vi "Samp.vi"() -> ()   [LabVIEW 2020]
panel:
  out "subarray":dbl[](array[numeric])
  out "Array 2":i32[](array[numeric])
  out "Array":i32[](array[numeric])
  out "x*y":dbl
  out "Waveform Graph":cluster{i32, dbl, i32[]}(graph)
  in  "stop":bool
  out "x":i32
  out "min index(es)":i32
  out "min value":i32
  out "max index(es)":i32
  out "max value":i32
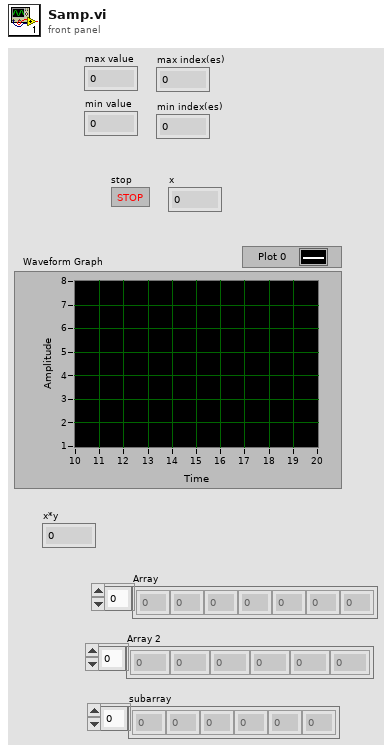
[diagram p1: front panel]
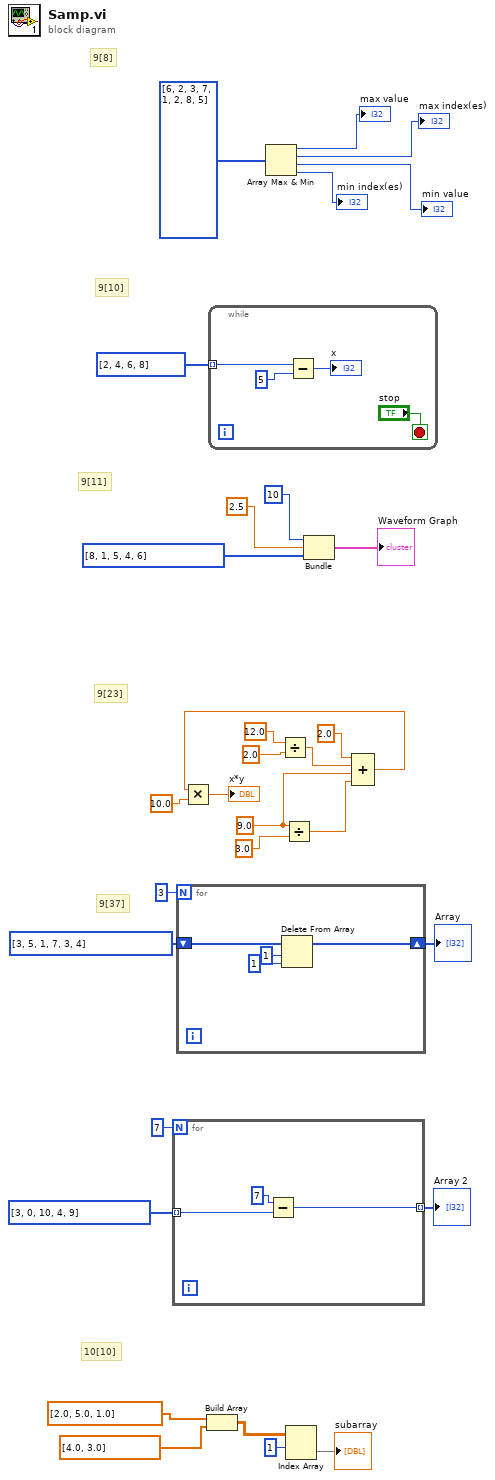
[diagram p0: block diagram]
diagram:
  w12 = 9.0
  # "10[10]"
  # "9[37]"
  # "9[23]"
  # "9[11]"
  # "9[10]"
  # "9[8]"
  n1 = for {
    N: 7 -> [_]
    tunnel: i32[] [3, 0, 10, 4, 9] -> [w33] mode=indexing
    tunnel: [w32] -> w6 mode=indexing
    n2 = Subtract(x=7, y=w33) -> (x-y=w32:i32)
  }
  "Array 2" <- w6
  n3 = for {
    N: 3 -> [_]
    shift-right: [w35] -> w10
    shift-left: i32[] [3, 5, 1, 7, 3, 4] -> [w38]
    n4 = Delete From Array(array=w38, length=1, index=1) -> (array with subset deleted=w35:i32[])  [unwired: 1 out]
  }
  "Array" <- w10
  n5 = Build Array(dbl[] [2.0, 5.0, 1.0], dbl[] [4.0, 3.0]) -> (w3:dbl[][])
  n6 = while {
    tunnel: i32[] [2, 4, 6, 8] -> [w42] mode=indexing
    stop <- "stop" stop-if-true
    n7 = Subtract(x=w42, y=5) -> (x-y=→"x":i32)
  }
  n8 = Array Max & Min(array=i32[] [6, 2, 3, 7, 1, 2, 8, 5]) -> (max value=→"max value":i32, max index (indices)=→"max index(es)":i32, min value=→"min value":i32, min index (indices)=→"min index(es)":i32)
  n9 = Divide(x=12.0, y=2.0) -> (x/y=w19:dbl)
  n10 = Divide(x=w12, y=3.0) -> (x/y=w13:dbl)
  n11 = Index Array(array=w3, index (row)=1) -> (element=→"subarray":dbl[])  [unwired: 1 in]
  n12 = Bundle(10, 2.5, i32[] [8, 1, 5, 4, 6]) -> (→"Waveform Graph":cluster{i32, dbl, i32[]})  [unwired: 1 in]
  n13 = Compound Arithmetic op=unknown(2.0, w19, w12, w13) -> (w14:dbl)
  n14 = Multiply(x=w14, y=10.0) -> (x*y=→"x*y":dbl)
